vi "mod_Narrow band low pass filter design (kaiser-sinc).vi"(0 "Maximum Decimation Factor (512)":enum16{"512", "1024", "2048", "4096"}(ring), 5 "Stop Band Attenuation (120 dB)":T1(ring)=enum."120 dB", 12 "Alias Protect in Final Transition? (T)":bool=TRUE) -> (4 "Filter Info":cluster{"h":dbl[], "Decimation":dbl} {"h" format="%.2f"; "Decimation" format="%.2f"})   [LabVIEW 2020, in "niAMT.lvlib"]
uses:
  <vilib>/addons/Modulation/niAMT.lvlib
panel:
  in  "debug?":bool
  out "frequency response":dbl[](graph)
  out "Estimated Taps":i32
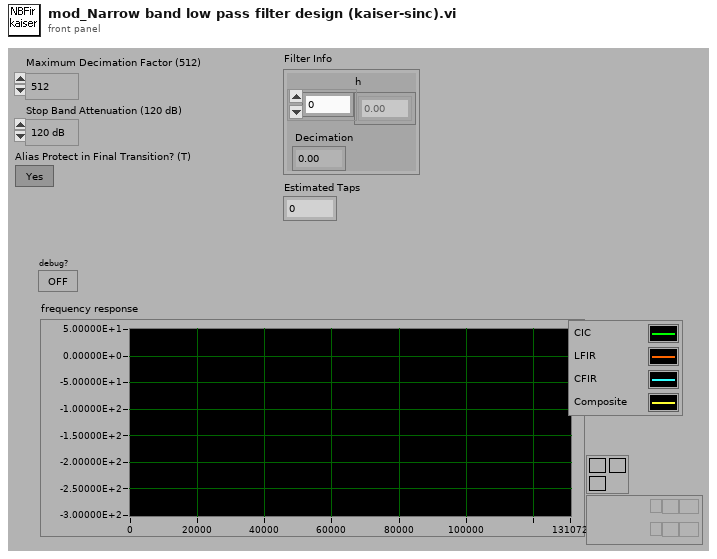
[diagram p1: front panel]
types:
  T1 = enum16{"48 dB", "60 dB", "72 dB", "84 dB", "96 dB", "120 dB"}
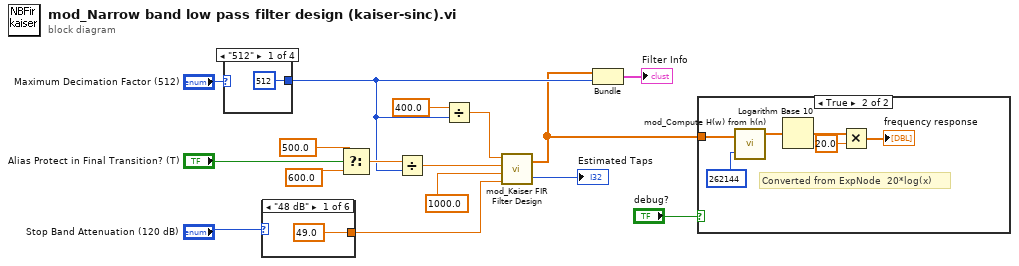
[diagram p0: block diagram]
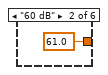
[diagram p3: hidden frame]
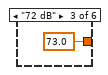
[diagram p4: hidden frame]
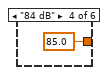
[diagram p5: hidden frame]
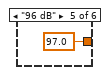
[diagram p6: hidden frame]
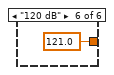
[diagram p7: hidden frame]
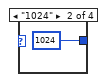
[diagram p8: hidden frame]
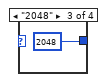
[diagram p9: hidden frame]
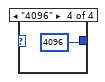
[diagram p10: hidden frame]
diagram:
  n1 = case shown="\"512\"" "Maximum Decimation Factor (512)" {
    tunnel: [512 1024 2048 4096] -> w4
    frame "512" {
    }
    frame "1024" {
    }
    frame "2048" {
    }
    frame "4096" {
    }
  }
  n2 = case shown="\"48 dB\"" "Stop Band Attenuation (120 dB)" {
    tunnel: [49.0 61.0 73.0 85.0 97.0 121.0] -> w14
    frame "48 dB" {
    }
    frame "60 dB" {
    }
    frame "72 dB" {
    }
    frame "84 dB" {
    }
    frame "96 dB" {
    }
    frame "120 dB" {
    }
  }
  n3 = Select(t=500.0 ("high cutoff freq: fh"), s="Alias Protect in Final Transition? (T)", f=600.0 ("high cutoff freq: fh")) -> (s? t:f=w13:dbl)
  n4 = Divide(x=w13, y=w4) -> (x/y=w5:dbl)
  n5 = Divide(x=400.0 ("low cutoff freq: fl"), y=w4) -> (x/y=w6:dbl)
  n6 = call <vilib>:"mod_Kaiser FIR Filter Design.vi"("Stop Attenuation"=w14, "sampling freq: fs"=1000.0, "high cutoff freq: fh"=w5, "low cutoff freq: fl"=w6) -> ("Estimated Taps"=→"Estimated Taps":i32, "h"=w2:dbl[])
  n7 = Bundle("h"=w2, w4) -> (→"Filter Info":cluster{"h":dbl[], i32})  [unwired: 1 out]
  n8 = case shown="True" "debug?" {
    tunnel: w2 -> [_ w32]
    frame False {
    }
    frame True {
      # "Converted from ExpNode \t20*log(x)"
      n9 = call <vilib>:"mod_Compute H(w) from h(n).vi"("h"=w32, "FFT size"=262144) -> ("Mag H(w)"=w28:dbl[])  [unwired: 2 out]
      n10 = Logarithm Base 10(1:w28) -> (0:w29:dbl[])
      n11 = Multiply(x=w29, y=20.0) -> (x*y=→"frequency response":dbl[])
    }
  }
